vi "OPC UA Secure Read Client2.vi"() -> ()   [LabVIEW 2017]
uses:
  <vilib>/OPCUA/NI OPC UA Client.lvlib
  <vilib>/OPCUA/controls/NodeId.ctl
  <vilib>/OPCUA/controls/NodeIds.ctl
  <vilib>/OPCUA/client/Multiple Write Variant.vi
panel:
  in  "Device.Node.Set Point":dbl
  in  "stop":bool
  in  "trusted server certificates":path[](array[path])
  in  "client certificate file":path
  in  "server endpoint URL":string
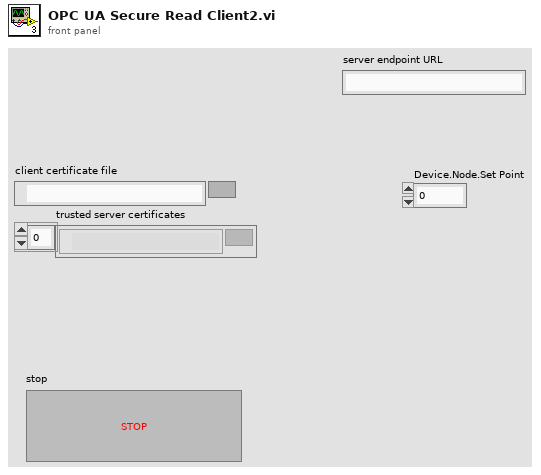
[diagram p1: front panel]
types:
  T1 = typedef "NodeIds.ctl" = T2[]
  T2 = typedef "NodeId.ctl" = string
  T3 = typedef "OPC UA Client Refnum.ctl" = refnum<k21>
  T4 = typedef "Subscription ID.ctl" = u32
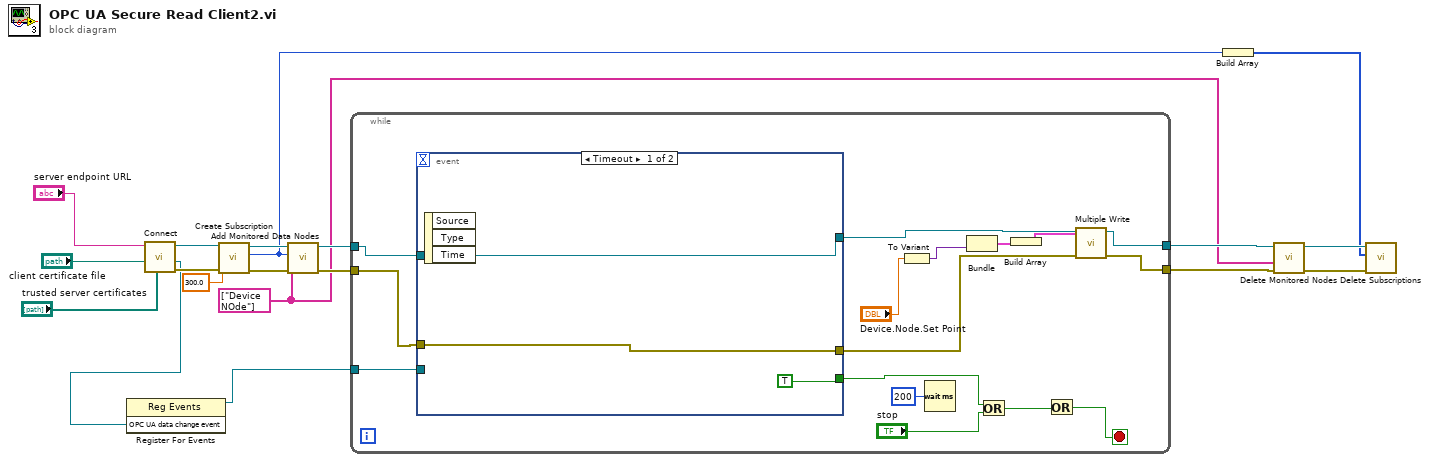
[diagram p0: block diagram]
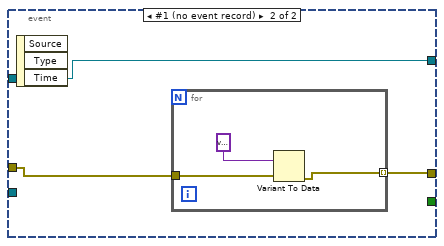
[diagram p2: hidden frame]
diagram:
  w1 = T1 ["Device NOde"] ("node IDs")
  n1 = call <vilib>:"Connect.vi"("trusted server certificates"="trusted server certificates", "client certificate file"="client certificate file", "server endpoint URL"="server endpoint URL") -> ("error out"=w15:errorcluster, "OPC UA data change event"=w13:refnum<user-event>, "OPC UA client refnum out"=w16:T3)  [unwired: 6 in]
  n2 = register-events(w13) -> (reference out=w12:refnum<event-registration>)  [unwired: 2 in, 1 out]
  n3 = call <vilib>:"Create Subscription.vi"("error in (no error)"=w15, "publishing interval (1000 ms)"=300.0, "OPC UA client refnum in"=w16) -> ("error out"=w10:errorcluster, "subscription ID out"=w2:T4, "OPC UA client refnum out"=w11:T3)  [unwired: 4 in, 2 out]
  n4 = call <vilib>:"Add Monitored Data Nodes.vi"("error in (no error)"=w10, "node IDs"=w1, "subscription ID in"=w2, "OPC UA client refnum in"=w11) -> ("error out"=w8:errorcluster, "OPC UA client refnum out"=w9:T3)  [unwired: 4 in, 2 out]
  n5 = while {
    tunnel: [w28] -> w7
    tunnel: [w25] -> w6
    tunnel: w12 -> [w27]
    tunnel: w9 -> [w33]
    tunnel: w8 -> [w34]
    stop <- w30 stop-if-true
    n6 = event shown="[0] Timeout" {
      selector: _ -> [_ _]
      dyn-events: _ -> [_ _]
      timeout: _ -> [_ _]
      tunnel: w34 -> [w37 w39]
      tunnel: [w37 w40] -> w26
      tunnel: w33 -> [w38 w41]
      tunnel: [w38 w41] -> w29
      tunnel: w27 -> [_ _]
      tunnel: [TRUE _] -> w20
      event Timeout {
        n7 = event-data() -> ()  [unwired: 1 in, 3 out]
      }
      event #1 (no event record) {
        n8 = event-data() -> ()  [unwired: 1 in, 3 out]
        n9 = for {
          tunnel: w39 -> [w44]
          tunnel: [w42] -> w40 mode=indexing
          n10 = Variant To Data(error in=w44, type=variant) -> (error out=w42:errorcluster)  [unwired: 1 in, 1 out]
        }
      }
    }
    n11 = To Variant(anything="Device.Node.Set Point") -> (Variant=w23:variant)
    n12 = Wait (ms)(milliseconds to wait=u32 200) -> ()  [unwired: 1 out]
    n13 = Bundle("Variant"=w23) -> (w22:cluster{void, "Variant":variant})  [unwired: 2 in]
    n14 = Or(x=w20, y="stop") -> (x .or. y?=w31:bool)
    n15 = Build Array(w22) -> (w21:cluster{void, "Variant":variant}[])
    n16 = Or(y=w31) -> (x .or. y?=w30:bool)  [unwired: 1 in]
    n17 = call-poly <vilib>:"Multiple Write.vi"("error in (no error)"=w26, "requests"=w21, "OPC UA client refnum in"=w29) -> ("error out"=w25:errorcluster, "OPC UA client refnum out"=w28:T3)  [unwired: 5 in, 2 out]
  }
  n18 = Build Array(w2) -> (w3:T4[])
  n19 = call <vilib>:"Delete Monitored Nodes.vi"("error in (no error)"=w6, "node IDs"=w1, "OPC UA client refnum in"=w7) -> ("error out"=w4:errorcluster, "OPC UA client refnum out"=w5:T3)  [unwired: 4 in, 3 out]
  n20 = call <vilib>:"Delete Subscriptions.vi"("error in (no error)"=w4, "subscription IDs"=w3, "OPC UA client refnum in"=w5) -> ()  [unwired: 6 in, 3 out]
